vi "tempset.vi"() -> ()   [LabVIEW 2010]
panel:
  in  "mode (0)":i16
  out "Numeric":dbl
  out "error out 2":errorcluster
  in  "Wait/s":dbl format="%.2f"
  in  "error in (no error)":errorcluster
  in  "Voltage":dbl format="%.2f"
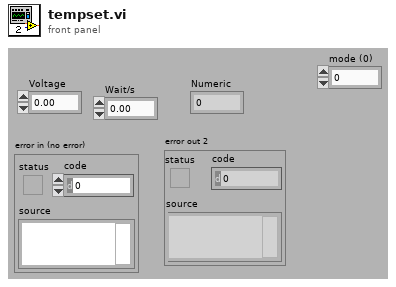
[diagram p1: front panel]
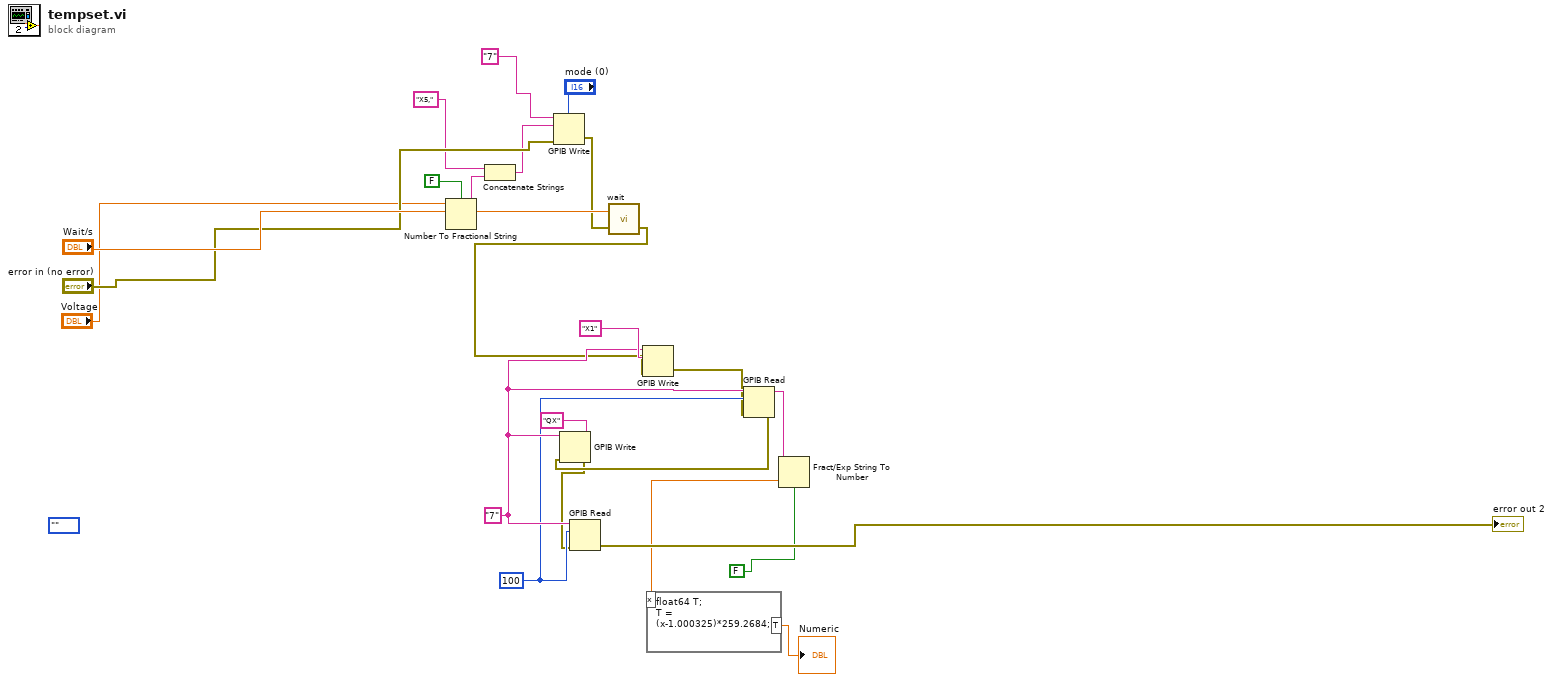
[diagram p0: block diagram]
diagram:
  w15 = 100
  w17 = "7"
  (unwired) enum16{""}.""
  n1 = Number To Fractional String(use system decimal point (T)=FALSE, number="Voltage") -> (F-format string=w5:string)  [unwired: 2 in]
  n2 = Concatenate Strings("X5,", w5) -> (w3:string)
  n3 = GPIB Write(0:"7", 1:w3, 2:"mode (0)", 3:"error in (no error)") -> (6:w6:errorcluster)  [unwired: 1 in, 1 out]
  n4 = call "wait.vi"("error in"=w6, "Wartezeit in Sek"="Wait/s") -> ("error out"=w1:errorcluster)  [unwired: 1 in]
  n5 = GPIB Write(0:w17, 1:"X1", 3:w1) -> (6:w14:errorcluster)  [unwired: 2 in, 1 out]
  n6 = GPIB Read(0:w17, 1:w15, 3:w14) -> (5:w12:string, 7:w11:errorcluster)  [unwired: 2 in, 1 out]
  n7 = GPIB Write(0:w17, 1:"QX", 3:w11) -> (6:w10:errorcluster)  [unwired: 2 in, 1 out]
  n8 = GPIB Read(0:w17, 1:w15, 3:w10) -> (7:→"error out 2":errorcluster)  [unwired: 2 in, 2 out]
  n9 = Fract/Exp String To Number(use system decimal point (T)=FALSE, string=w12) -> (number=w13:dbl)  [unwired: 2 in, 1 out]
  n10 = formula code="float64 T;\nT = (x-1.000325)*259.2684;"("x"=w13) -> ("T"=→"Numeric":dbl)
